vi "uPolicy_TopicIsRelevant.vi"(8 "error in (no error)":errorcluster, 10 "Observed Topic (Lower Case)":string, 11 "hasPrefix_All in":refnum<class "hasPrefix.lvclass">) -> (0 "error out":errorcluster, 2 "Relevant?":bool, 3 "hasPrefix_All out":refnum<class "hasPrefix.lvclass">)   [LabVIEW 2021, in "uFramework_pack_uPolicy.lvlib" / "hasPrefix.lvclass"]
uses:
  hasPrefix.lvclass
  hasPrefix.lvclass/hasPrefix.ctl
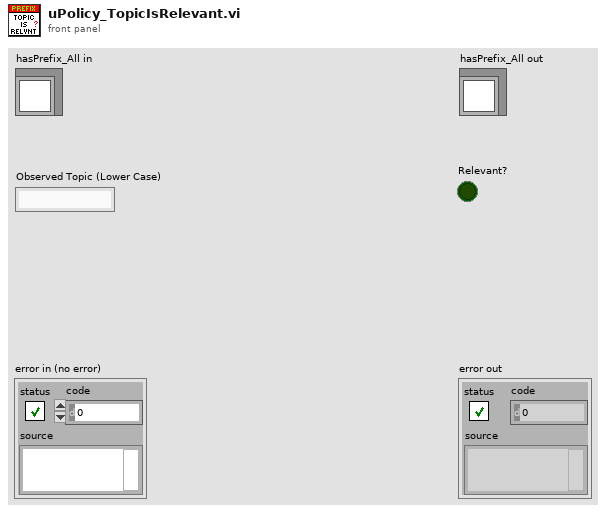
[diagram p1: front panel]
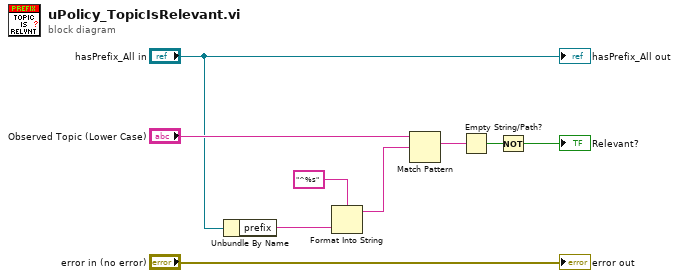
[diagram p0: block diagram]
diagram:
  n1 = Unbundle By Name("hasPrefix_All in") -> ("prefix"=w6:string)
  n2 = Format Into String(format string="^%s", w6) -> (resulting string=w4:string)  [unwired: 2 in, 1 out]
  n3 = Match Pattern(string="Observed Topic (Lower Case)", regular expression=w4) -> (match substring=w3:string)  [unwired: 1 in, 3 out]
  n4 = Empty String/Path?(string/path=w3) -> (empty?=w2:bool)
  n5 = Not(x=w2) -> (.not. x?=→"Relevant?":bool)
  "error out" <- "error in (no error)"
  "hasPrefix_All out" <- "hasPrefix_All in"
